vi "Criteri salvataggii report.vi"(11 "Default?":bool=TRUE) -> (2 "ANNULLA?":bool, 3 "OUT":string[](array[string]))   [LabVIEW 2019]
uses:
  Global percorso impostazioni.vi
  <vilib>/Utility/file.llb/Read Delimited Spreadsheet (string).vi
  <vilib>/addons/database/NI_Database_API.lvlib
panel:
  in  "SCOPO":string(combo)
  in  "Annulla":bool
  in  "Tab Control":T1(tab)
  in  "Percorso salvataggio gestionale":path
  in  "Percorso salvataggio report standard":path
  in  "percorso inserito":bool
  in  "elimina da nome":bool
  in  "inserisci separatore":bool
  in  "Carattere/stringa di separazione":string
  in  "Nome report":i32(listbox)
  in  "inserisci campo nome":bool
  in  "Lista campi 2":i32(listbox) caption="Lista campi"
  in  "OK Button":bool
  # "DEFAULT"
  # "INSERISCI I PERCORSI DI SALVATAGGIO"
  # "CREA NOME DI SALVAGGIO REPORT"
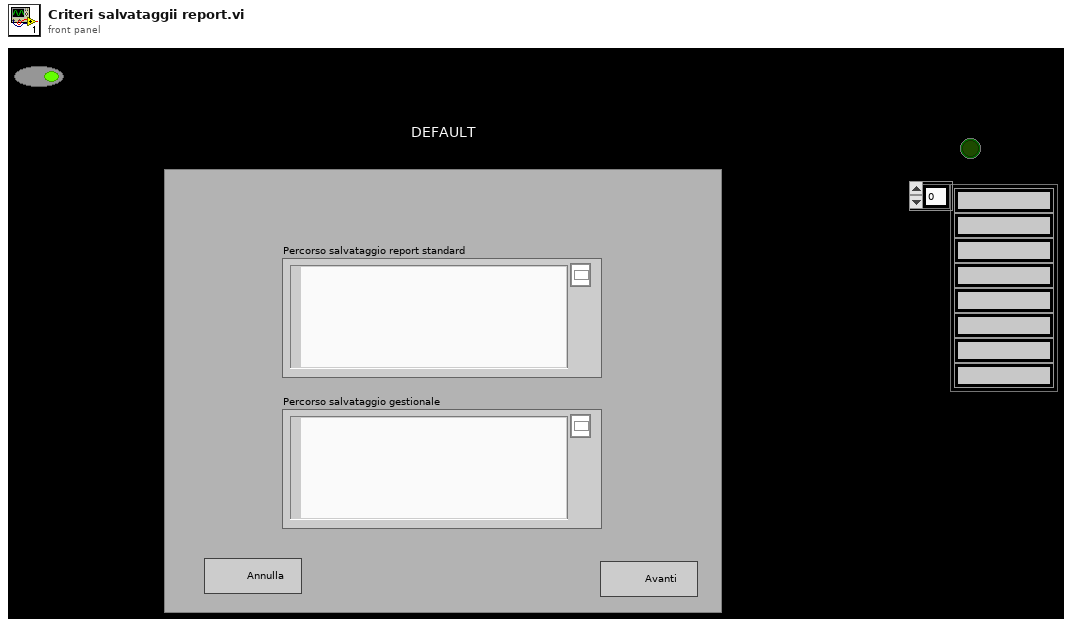
[diagram p1: front panel]
types:
  T1 = enum32{"inserimento percorso", "Nome di default"}
  T2 = typedef "NI_Database_API.lvlib/Conn ObjectReference.ctl" = refnum<k1>
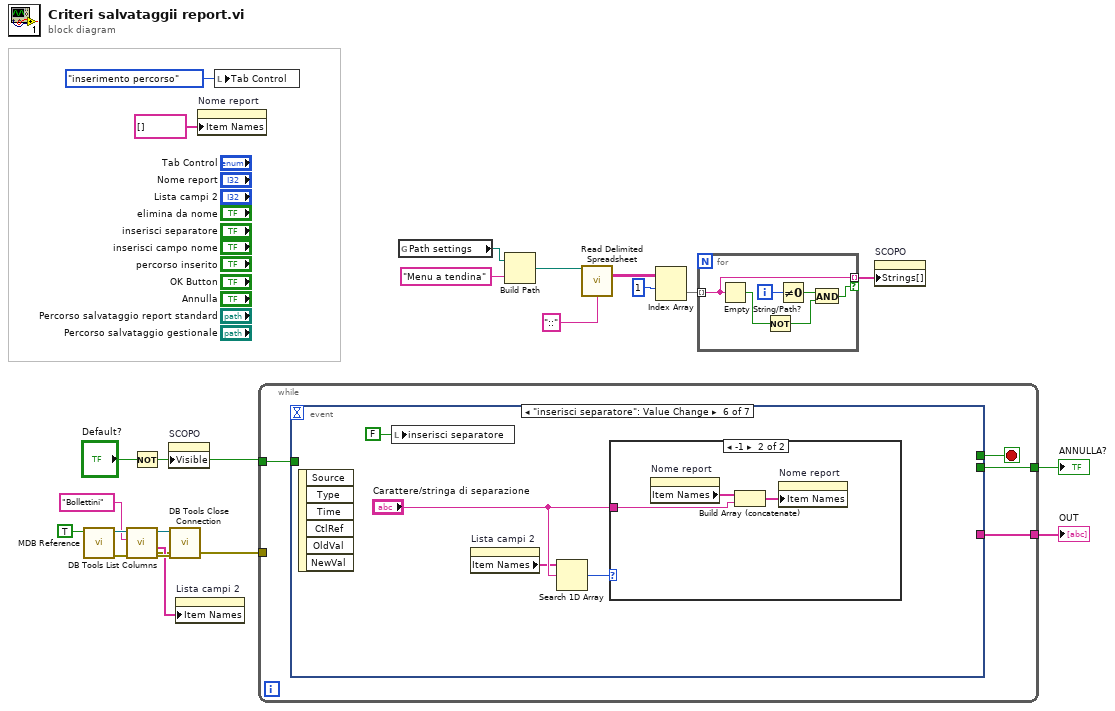
[diagram p0: block diagram]
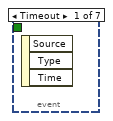
[diagram p2: hidden frame]
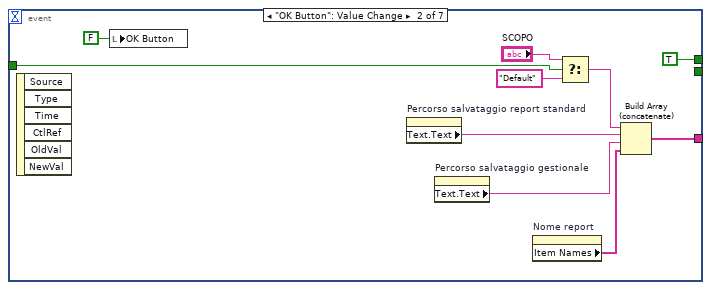
[diagram p3: hidden frame]
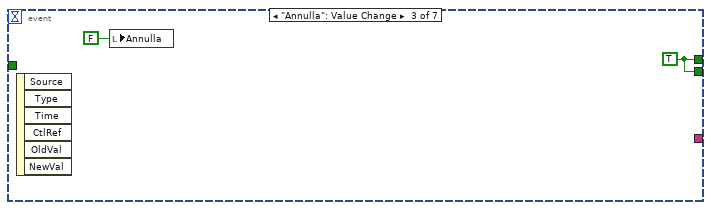
[diagram p4: hidden frame]
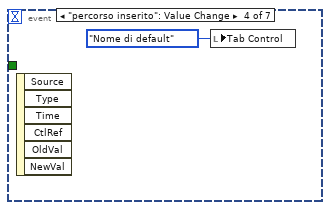
[diagram p5: hidden frame]
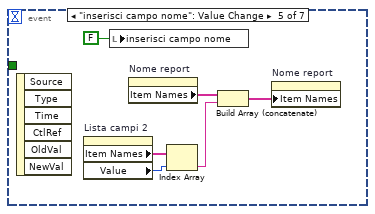
[diagram p6: hidden frame]
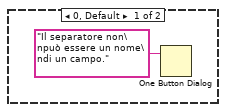
[diagram p7: hidden frame]
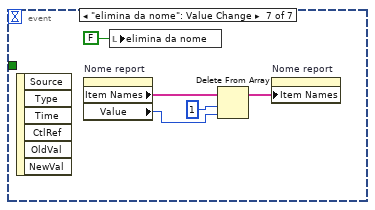
[diagram p8: hidden frame]
diagram:
  n1 = call "MDB Reference.vi"("Collaudi T/motori F"=TRUE) -> ("error out"=w5:errorcluster, "Refnum out"=w6:T2)  [unwired: 8 in, 1 out]
  n2 = call <vilib>:"DB Tools List Columns.vi"("error in (no error)"=w5, "table"="Bollettini", "connection reference"=w6) -> ("error out"=w7:errorcluster, "columns"=w3:string[], "connection reference out"=w8:T2)  [unwired: 1 in, 1 out]
  n3 = Not(x="Default?") -> (.not. x?=w9:bool)
  n4 = property on="SCOPO" class="CmbBox"("Visible"=w9) -> ()  [unwired: 2 in, 2 out]
  n5 = call <vilib>:"DB Tools Close Connection.vi"("error in (no error)"=w7, "connection reference"=w8) -> ("error out"=w2:errorcluster)  [unwired: 5 in]
  n6 = property on="Lista campi 2" class="LstBox (strict)"("Item Names"=w3) -> ()  [unwired: 2 in, 2 out]
  n7 = property on="Nome report" class="LstBox (strict)"("Item Names"=string[] []) -> ()  [unwired: 2 in, 2 out]
  n8 = local write "Tab Control"(T1."inserimento percorso" ("Tab Control")) -> ()
  n9 = while {
    tunnel: [w25] -> w22
    tunnel: [w24] -> w21
    tunnel: w9 -> [w23]
    tunnel: w2 -> [_]
    stop <- w26 stop-if-true
    n10 = event shown="[5] \"inserisci separatore\": Value Change" {
      selector: _ -> [_ _ _ _ _ _ _]
      dyn-events: _ -> [_ _ _ _ _ _ _]
      timeout: _ -> [_ _ _ _ _ _ _]
      tunnel: [_ TRUE w38 _ _ _ _] -> w26
      tunnel: [_ w34 _ _ _ _ _] -> w25
      tunnel: [_ _ w38 _ _ _ _] -> w24
      tunnel: w23 -> [_ w32 _ _ _ _ _]
      event Timeout {
        n11 = event-data() -> ()  [unwired: 1 in, 3 out]
      }
      event "OK Button": Value Change {
        n12 = event-data() -> ()  [unwired: 1 in, 6 out]
        n13 = local write "OK Button"(FALSE ("OK Button")) -> ()
        n14 = property on="Percorso salvataggio report standard" class="Path"() -> ("Text.Text"=w35:string)  [unwired: 2 in, 2 out]
        n15 = property on="Percorso salvataggio gestionale" class="Path"() -> ("Text.Text"=w27:string)  [unwired: 2 in, 2 out]
        n16 = property on="Nome report" class="LstBox (strict)"() -> ("Item Names"=w28:string[])  [unwired: 2 in, 2 out]
        n17 = Select(t="SCOPO", s=w32, f="Default") -> (s? t:f=w30:string)
        n18 = Build Array (concatenate)(w30, w35, w27, w28) -> (w34:string[])
      }
      event "Annulla": Value Change {
        w38 = TRUE
        n19 = event-data() -> ()  [unwired: 1 in, 6 out]
        n20 = local write "Annulla"(FALSE ("Annulla")) -> ()
      }
      event "percorso inserito": Value Change {
        n21 = event-data() -> ()  [unwired: 1 in, 6 out]
        n22 = local write "Tab Control"(T1."Nome di default" ("Tab Control")) -> ()
      }
      event "inserisci campo nome": Value Change {
        n23 = event-data() -> ()  [unwired: 1 in, 6 out]
        n24 = property on="Lista campi 2" class="LstBox (strict)"() -> ("Item Names"=w45:string[], "Value"=w44:i32)  [unwired: 2 in, 2 out]
        n25 = local write "inserisci campo nome"(FALSE ("inserisci campo nome")) -> ()
        n26 = property on="Nome report" class="LstBox (strict)"() -> ("Item Names"=w43:string[])  [unwired: 2 in, 2 out]
        n27 = Index Array(array=w45, index=w44) -> (element=w42:string)
        n28 = Build Array (concatenate)(w43, w42) -> (w41:string[])
        n29 = property on="Nome report" class="LstBox (strict)"("Item Names"=w41) -> ()  [unwired: 2 in, 2 out]
      }
      event "inserisci separatore": Value Change {
        n30 = event-data() -> ()  [unwired: 1 in, 6 out]
        n31 = local write "inserisci separatore"(FALSE ("inserisci separatore")) -> ()
        n32 = property on="Lista campi 2" class="LstBox (strict)"() -> ("Item Names"=w47:string[])  [unwired: 2 in, 2 out]
        n33 = Search 1D Array(1D array=w47, element="Carattere/stringa di separazione") -> (index of element=w46:i32)  [unwired: 1 in]
        n34 = case shown="-1" w46 {
          tunnel: "Carattere/stringa di separazione" -> [_ w51]
          frame 0, Default {
            n35 = One Button Dialog(message="Il separatore non\npuò essere un nome\ndi un campo.") -> ()  [unwired: 1 in, 1 out]
          }
          frame -1 {
            n36 = property on="Nome report" class="LstBox (strict)"() -> ("Item Names"=w53:string[])  [unwired: 2 in, 2 out]
            n37 = Build Array (concatenate)(w53, w51) -> (w52:string[])
            n38 = property on="Nome report" class="LstBox (strict)"("Item Names"=w52) -> ()  [unwired: 2 in, 2 out]
          }
        }
      }
      event "elimina da nome": Value Change {
        n39 = event-data() -> ()  [unwired: 1 in, 6 out]
        n40 = property on="Nome report" class="LstBox (strict)"() -> ("Item Names"=w58:string[], "Value"=w57:i32)  [unwired: 2 in, 2 out]
        n41 = local write "elimina da nome"(FALSE ("elimina da nome")) -> ()
        n42 = Delete From Array(array=w58, length=1, index=w57) -> (array with subset deleted=w55:string[])  [unwired: 1 out]
        n43 = property on="Nome report" class="LstBox (strict)"("Item Names"=w55) -> ()  [unwired: 2 in, 2 out]
      }
    }
  }
  "OUT" <- w22
  "ANNULLA?" <- w21
  n44 = global read "Global percorso impostazioni.vi" "Path settings"() -> (w16:path)
  n45 = Build Path(base path=w16, name or relative path="Menu a tendina") -> (appended path=w18:path)
  n46 = call-poly <vilib>:"Read Delimited Spreadsheet.vi"("file path (dialog if empty)"=w18, "delimiter (\\t)"="::" ("delimiter (\\t)")) -> ("all rows"=w15:string[][])  [unwired: 8 in, 5 out]
  n47 = Index Array(array=w15, index (row)=1) -> (element=w13:string[])  [unwired: 1 in]
  n48 = for {
    tunnel: w13 -> [w64] mode=indexing
    tunnel: [w64] -> w12 mode=indexing if=w61
    i -> [w60]
    n49 = Empty String/Path?(string/path=w64) -> (empty?=w63:bool)
    n50 = Not(x=w63) -> (.not. x?=w62:bool)
    n51 = Not Equal To 0?(x=w60) -> (x != 0?=w59:bool)
    n52 = And(x=w59, y=w62) -> (x .and. y?=w61:bool)
  }
  n53 = property on="SCOPO" class="CmbBox"("Strings[]"=w12) -> ()  [unwired: 2 in, 2 out]
